vi "Fastseq_slot_to_order.vi"(1 "index":i32, 2 "Type":i32, 3 "data1":dbl, 4 "data2":dbl) -> (0 "Order":u64)   [LabVIEW 2013]
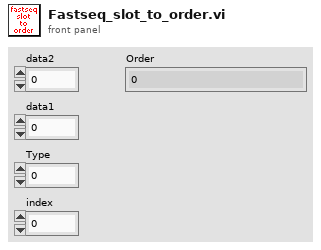
[diagram p1: front panel]
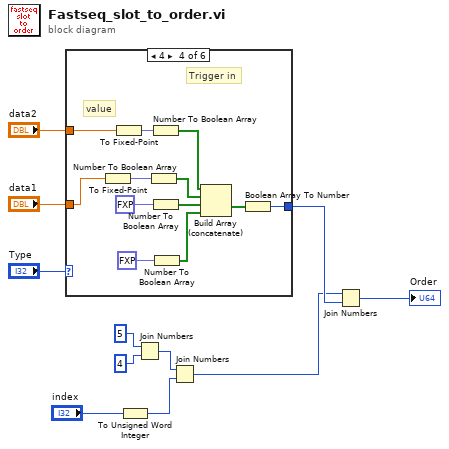
[diagram p0: block diagram]
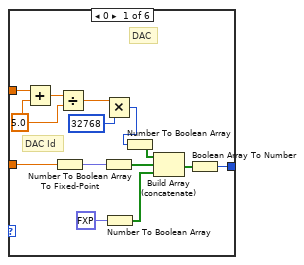
[diagram p2: hidden frame]
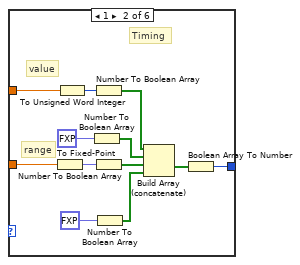
[diagram p3: hidden frame]
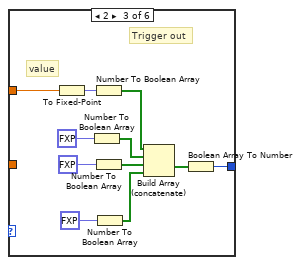
[diagram p4: hidden frame]
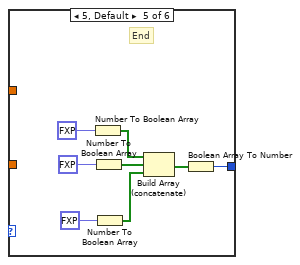
[diagram p5: hidden frame]
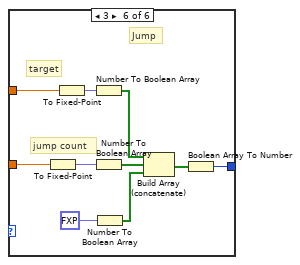
[diagram p6: hidden frame]
diagram:
  n1 = case shown="4" "Type" {
    tunnel: "data1" -> [w25 w37 _ w50 _ w71]
    tunnel: "data2" -> [w17 w36 w48 w60 _ w78]
    tunnel: [w18 w29 w43 w54 w64 w72] -> w2
    frame 0 {
      w15 = 5.0 ("y")
      # "DAC Id"
      # "DAC"
      n2 = Add(x=w17, y=w15) -> (x+y=w16:dbl)
      n3 = To Fixed-Point(number=w25) -> (fixed-point=w23:fxp<+,6,6>)  [unwired: 1 in]
      n4 = Divide(x=w16, y=w15) -> (x/y=w14:dbl)
      n5 = Multiply(x=w14, y=u16 32768) -> (x*y=w12:u16)
      n6 = Number To Boolean Array(number=w23) -> (Boolean array=w20:bool[])
      n7 = Number To Boolean Array(number=fxp<+,2,2> 0.0 ("hi")) -> (Boolean array=w21:bool[])
      n8 = Number To Boolean Array(number=w12) -> (Boolean array=w22:bool[])
      n9 = Build Array (concatenate)(w22, w20, w21) -> (w19:bool[])
      n10 = Boolean Array To Number(Boolean array=w19) -> (number=w18:u32)
    }
    frame 1 {
      # "value"
      # "range"
      # "Timing"
      n11 = To Fixed-Point(number=w37) -> (fixed-point=w34:fxp<+,2,2>)  [unwired: 1 in]
      n12 = To Unsigned Word Integer(number=w36) -> (unsigned 16bit integer=w33:u16)
      n13 = Number To Boolean Array(number=fxp<+,4,4> 0.0 ("hi")) -> (Boolean array=w26:bool[])
      n14 = Number To Boolean Array(number=w33) -> (Boolean array=w28:bool[])
      n15 = Number To Boolean Array(number=w34) -> (Boolean array=w31:bool[])
      n16 = Number To Boolean Array(number=fxp<+,2,2> 1.0 ("hi")) -> (Boolean array=w32:bool[])
      n17 = Build Array (concatenate)(w28, w26, w31, w32) -> (w30:bool[])
      n18 = Boolean Array To Number(Boolean array=w30) -> (number=w29:u32)
    }
    frame 2 {
      # "value"
      # "Trigger out"
      n19 = To Fixed-Point(number=w48) -> (fixed-point=w46:fxp<+,10,10>)  [unwired: 1 in]
      n20 = Number To Boolean Array(number=fxp<+,10,10> 0.0 ("hi")) -> (Boolean array=w40:bool[])
      n21 = Number To Boolean Array(number=w46) -> (Boolean array=w42:bool[])
      n22 = Number To Boolean Array(number=fxp<+,2,2> 0.0) -> (Boolean array=w44:bool[])
      n23 = Number To Boolean Array(number=fxp<+,2,2> 2.0 ("hi")) -> (Boolean array=w45:bool[])
      n24 = Build Array (concatenate)(w42, w40, w44, w45) -> (w38:bool[])
      n25 = Boolean Array To Number(Boolean array=w38) -> (number=w43:u32)
    }
    frame 4 {
      # "value"
      # "Trigger in"
      n26 = To Fixed-Point(number=w50) -> (fixed-point=w49:fxp<+,10,10>)  [unwired: 1 in]
      n27 = To Fixed-Point(number=w60) -> (fixed-point=w58:fxp<+,10,10>)  [unwired: 1 in]
      n28 = Number To Boolean Array(number=w49) -> (Boolean array=w52:bool[])
      n29 = Number To Boolean Array(number=w58) -> (Boolean array=w53:bool[])
      n30 = Number To Boolean Array(number=fxp<+,2,2> 1.0) -> (Boolean array=w56:bool[])
      n31 = Number To Boolean Array(number=fxp<+,2,2> 2.0 ("hi")) -> (Boolean array=w57:bool[])
      n32 = Build Array (concatenate)(w53, w52, w56, w57) -> (w55:bool[])
      n33 = Boolean Array To Number(Boolean array=w55) -> (number=w54:u32)
    }
    frame 5, Default {
      # "End"
      n34 = Number To Boolean Array(number=fxp<+,20,20> 0.0) -> (Boolean array=w61:bool[])
      n35 = Number To Boolean Array(number=fxp<+,2,2> 2.0) -> (Boolean array=w66:bool[])
      n36 = Number To Boolean Array(number=fxp<+,2,2> 2.0 ("hi")) -> (Boolean array=w67:bool[])
      n37 = Build Array (concatenate)(w61, w66, w67) -> (w65:bool[])
      n38 = Boolean Array To Number(Boolean array=w65) -> (number=w64:u32)
    }
    frame 3 {
      # "jump count"
      # "target"
      # "Jump"
      n39 = To Fixed-Point(number=w71) -> (fixed-point=w70:fxp<+/-,10,10>)  [unwired: 1 in]
      n40 = To Fixed-Point(number=w78) -> (fixed-point=w76:fxp<+/-,12,12>)  [unwired: 1 in]
      n41 = Number To Boolean Array(number=w76) -> (Boolean array=w69:bool[])
      n42 = Number To Boolean Array(number=w70) -> (Boolean array=w74:bool[])
      n43 = Number To Boolean Array(number=fxp<+,2,2> 3.0 ("hi")) -> (Boolean array=w75:bool[])
      n44 = Build Array (concatenate)(w69, w74, w75) -> (w73:bool[])
      n45 = Boolean Array To Number(Boolean array=w73) -> (number=w72:u32)
    }
  }
  n46 = To Unsigned Word Integer(number="index") -> (unsigned 16bit integer=w6:u16)
  n47 = Join Numbers(hi=u8 5, lo=u8 4) -> ((hi.lo)=w7:u16)
  n48 = Join Numbers(hi=w7, lo=w6) -> ((hi.lo)=w1:u32)
  n49 = Join Numbers(hi=w1, lo=w2) -> ((hi.lo)=→"Order":u64)
